vi "WS1021 demo init.vi"() -> (0 "Error Out":errorcluster, 1 "De-embedding files":path[](array[path]), 2 "Toggle 8.lvclass":refnum<class "Toggle 8.lvclass">, 3 "Vector Network Analyzer.lvclass":refnum<class "Vector Network Analyzer.lvclass">, 4 "Cancelled":bool, 5 "VNA ports out":bool[](array[boolean])=[FALSE, FALSE, TRUE, TRUE], 6 "Error Limits 2":path)   [LabVIEW 2020]
uses:
  Instruments/Vector Network Analyzer/Vector Network Analyzer.lvclass
  C:/Sandbox/RF Bench/Source Code/WiSpry Test Framework/Instruments/Instrument.lvclass
  Devices/Toggle 8/Toggle 8.lvclass
  Instruments/Instrument.lvclass/Instrument.ctl
  Instruments/Instrument.lvclass
panel:
  in  "Error Limits":path
  in  "VNA ports":bool[](array[boolean])=[FALSE, FALSE, TRUE, TRUE]
  in  "WS1021 VISA address":refnum<visa-resource-name>
  in  "Cancel Button":bool
  in  "OK Button":bool
  in  "De-embedding files x2 & Virtual mode files x1":path[](array[path])=[path "", path "", path ""]
  in  "VNA model":u16(ring)=3 items=["Ag87xx", "CMT S2 S4", "FieldFox", "Keysight PNA", "PNA", "ZNB"]
  in  "VNA VISA address":refnum<visa-resource-name>
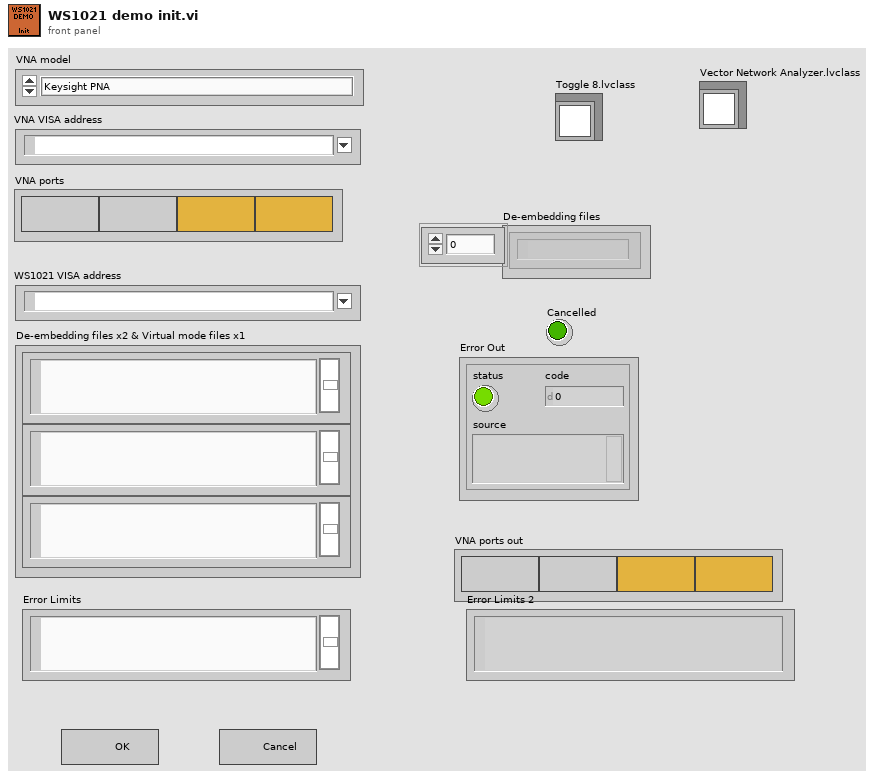
[diagram p1: front panel]
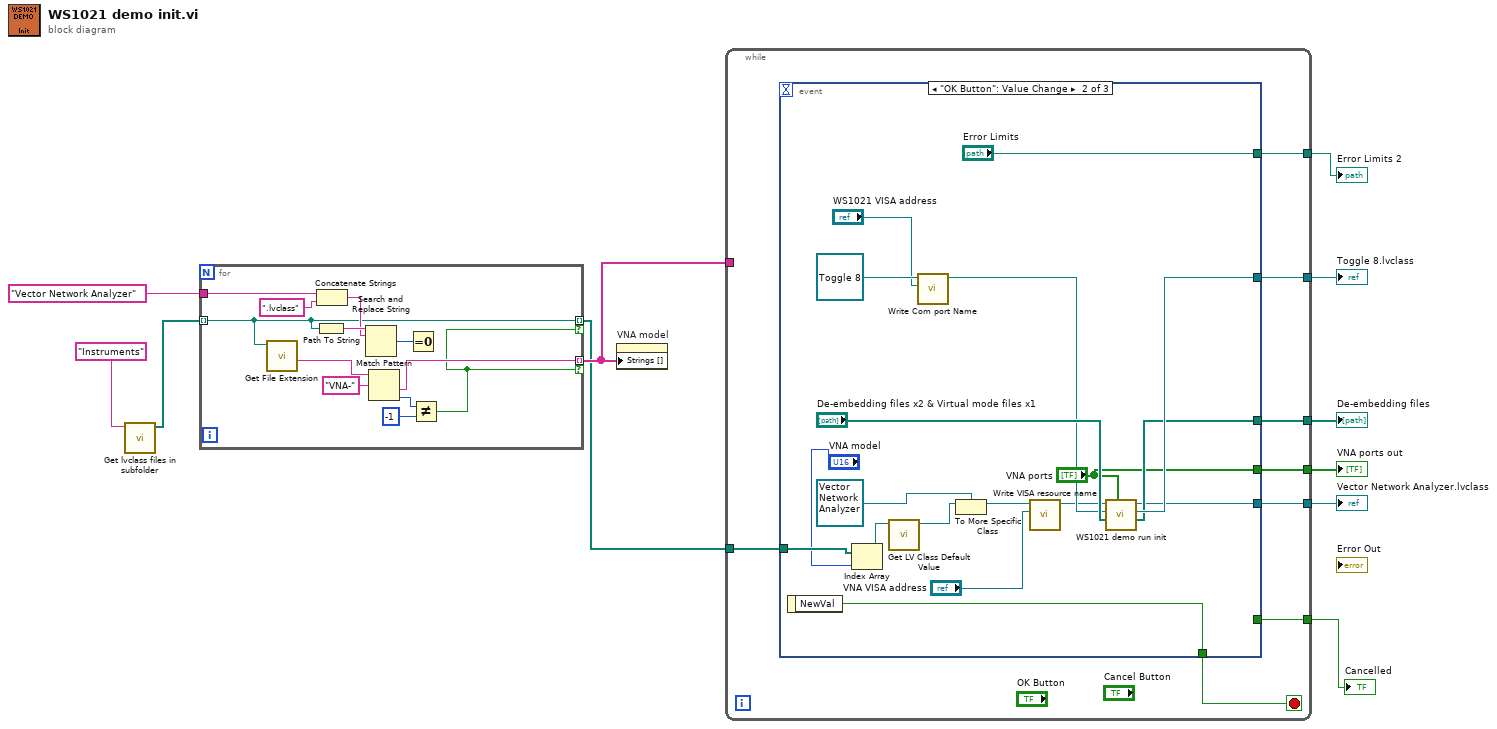
[diagram p0: block diagram]
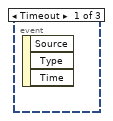
[diagram p2: hidden frame]
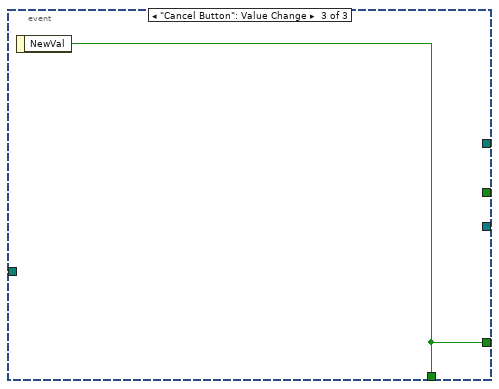
[diagram p3: hidden frame]
diagram:
  n1 = call "Get lvclass files in subfolder.vi"("Sub Folder"="Instruments") -> ("Found lvclass files"=w10:path[])  [unwired: 9 in, 1 out]
  n2 = for {
    tunnel: w10 -> [w18] mode=indexing
    tunnel: "Vector Network Analyzer" ("Sub Folder") -> [w21]
    tunnel: [w18] -> w4 mode=indexing if=w12
    tunnel: [w15] -> w8 mode=indexing if=w12
    n3 = call <vilib>:"Get File Extension.vi"("file"=w18) -> ("filename without extension"=w17:string)  [unwired: 6 in, 4 out]
    n4 = Path To String(path=w18) -> (string=w23:string)
    n5 = Concatenate Strings(w21, ".lvclass" ("string")) -> (w22:string)
    n6 = Search and Replace String(input string=w23, search string=w22) -> (number of replacements=w19:i32)  [unwired: 6 in, 3 out]
    n7 = Match Pattern(string=w17, regular expression="VNA-") -> (after substring=w15:string, offset past match=w14:i32)  [unwired: 1 in, 2 out]
    n8 = Equal To 0?(x=w19) -> ()  [unwired: 1 out]
    n9 = Not Equal?(x=w14, y=-1) -> (x != y?=w12:bool)
  }
  n10 = property on="VNA model" class="Ring (strict)"("Strings []"=w8) -> ()  [unwired: 2 in, 2 out]
  n11 = while {
    tunnel: w8 -> [_]
    tunnel: [w30] -> w7
    tunnel: [w29] -> w6
    tunnel: [w28] -> w5
    tunnel: w4 -> [w27]
    tunnel: [w26] -> w3
    tunnel: [w25] -> w2
    tunnel: [w24] -> w1
    stop <- w31 stop-if-true
    n12 = event shown="[1] \"OK Button\": Value Change" {
      selector: _ -> [_ _ _]
      dyn-events: _ -> [_ _ _]
      timeout: _ -> [_ _ _]
      tunnel: [_ w49 w50] -> w31
      tunnel: [_ w42 _] -> w30
      tunnel: [_ w40 _] -> w29
      tunnel: [_ w43 _] -> w28
      tunnel: w27 -> [_ w39 _]
      tunnel: [_ "VNA ports" _] -> w26
      tunnel: [_ _ w50] -> w25
      tunnel: [_ "Error Limits" _] -> w24
      event Timeout {
        n13 = event-data() -> ()  [unwired: 1 in, 3 out]
      }
      event "OK Button": Value Change {
        n14 = event-data() -> ("NewVal"=w49:bool)  [unwired: 1 in]
        n15 = Index Array(array=w39, index="VNA model") -> (element=w37:path)
        n16 = call <vilib>:"Get LV Class Default Value.vi"("class path"=w37) -> ("object"=w36:refnum<class>)  [unwired: 9 in, 1 out]
        n17 = call-dynamic "Write Com port Name.vi"("Com port Name"="WS1021 VISA address", "Device in"=refnum<class "Toggle 8.lvclass"> refnum ("Toggle 8.lvclass")) -> ("Device out"=w44:refnum<class "Toggle 8.lvclass">)  [unwired: 9 in]
        n18 = To More Specific Class(target class=refnum<class "Vector Network Analyzer.lvclass"> refnum ("Vector Network Analyzer.lvclass"), reference=w36) -> (specific class reference=w34:refnum<class "Vector Network Analyzer.lvclass">)  [unwired: 1 in, 1 out]
        n19 = call "Write VISA resource name.vi"("VISA resource name"="VNA VISA address", "Instrument in"=w34) -> ("Instrument out"=w41:refnum<class "Vector Network Analyzer.lvclass">)  [unwired: 9 in]
        n20 = call "WS1021 demo run init.vi"("VNA ports"="VNA ports", "De-embedding files in"="De-embedding files x2 & Virtual mode files x1", "Toggle 8.lvclass in"=w44, "Vector Network Analyzer.lvclass in"=w41) -> ("De-embedding files"=w42:path[], "Toggle 8.lvclass"=w43:refnum<class "Toggle 8.lvclass">, "Vector Network Analyzer.lvclass"=w40:refnum<class "Vector Network Analyzer.lvclass">)  [unwired: 5 in]
      }
      event "Cancel Button": Value Change {
        n21 = event-data() -> ("NewVal"=w50:bool)  [unwired: 1 in]
      }
    }
  }
  "De-embedding files" <- w7
  "Vector Network Analyzer.lvclass" <- w6
  "Cancelled" <- w2
  "Toggle 8.lvclass" <- w5
  "VNA ports out" <- w3
  "Error Limits 2" <- w1
